vi "FineContrast_v3.0.vi"(3 "Contrast References":T4, 4 "Constrast Handles":T5, 5 "Scan Translation Exp Params":T2, 6 "Scan Translation Params":T6) -> (0 "Constrast Handles Out":T3, 1 "PZAPos & InstPow":dbl[][](array[numeric]), 2 "Spectra vs PZA":i32[][](array[numeric]))   [LabVIEW 2019]
uses:
  C:/Users/manip/Documents/Controle_Manip_2020/Thorlabs.MotionControl.KCube.SolenoidCLI.dll
  Thorlabs.MotionControl.KCube.SolenoidCLI.dll
  Light Field/lightfield-automation-labview/LightField Automation.lvclass
  TypeDefs/AcqMode.ctl
panel:
  out "KCube Shutter On?":bool
  out "range":dbl
  out "LinT End pos (mm)":dbl
  out "LinT Step Pos (mm)":dbl
  out "LinT Start Pos (mm)":dbl
  in  "ESP 301 error out":errorcluster
  in  "ESP 301 COM out":refnum<visa-resource-name>="COM1"
  out "ESP 301 error in":errorcluster
  out "ESP 301 COM":refnum<visa-resource-name>="COM1"
  in  "Photodiode error out":errorcluster {"code" format="%.0x"}
  out "Photodiode out":refnum<visa-resource-name>
  out "Scan Contrast Ctrls":refnum<vi>[](array[refnum])
  out "InstPow":dbl[](array[numeric])
  out "ExcPow_uW":dbl
  in  "ExcWL_nm":dbl
  out "Photodiode error in":errorcluster {"code" format="%.0x"}
  out "Photodiode in":refnum<visa-resource-name>
  out "WavelengthCalibration":dbl[](array[numeric])
  out "x+y":dbl
  out "Contrast Oscillations":refnum<vi>
  out "Contrast 1D Spectrum":refnum<vi>
  out "PZC out":string
  out "PZC error out":errorcluster
  out "Pause button":refnum<vi>
  in  "Stop button":refnum<vi>
  out "PZC Pos (usteps)":refnum<vi>
  out "PZA Positions":i32[](array[numeric])
  out "Contrast values":i32[](array[numeric])
  out "Contrast 1D Spectrum":cluster{dbl[], dbl[]}(graph) caption="64.0°"
  out "Contrast Oscillations":cluster{dbl[], dbl[]}(graph)
  out "LFA error out":errorcluster
  out "LFA out":refnum<class "LightField Automation.lvclass">
  in  "Acq Mode":T1=enum."Spectrum" caption="Mode :"
  in  "Acq Time (ms) 2":dbl=500.0 caption="Acq Time :" min=0.0 max=360000.0 step=50.0
  in  "Pause Contrast":bool
  in  "Stop Contrast":bool
  out "PZC Position Readout (usteps)":dbl caption="Readout (usteps)" min=-8.0 max=392.0
  out "Progess Bar":refnum<vi>
  out "Scan Spectrum Progess Bar":u8(slide) scale=0.0..100.0
  in  "LFA error in":errorcluster
  in  "LFA in":refnum<class "LightField Automation.lvclass">
  out "Shutter Device":refnum<vi>
  out "KCube Shutter Device Reference":refnum<k24>
  out "Shutter":refnum<vi>
  out "Shutter Ctrls":u16(ring)
  in  "CCD ROI":T7(ring)
  in  "Accumulations":dbl=1.0
  in  "LinTFine Step":dbl
  in  "LinTFine End":dbl
  in  "LinTFine Start":dbl
  # "ms"
types:
  T1 = typedef "AcqMode.ctl" = enum16{"Image", "Spectrum", "APD 1", "APD 2", "APD 1+2"}
  T2 = cluster{"Exposure Time (ms)":dbl, "Accumulations":dbl, "Excitation Wavelength (nm)":dbl, "Acq Mode":T1, "CCD ROI":enum16{"Custom ROI", "Full sensor", "Binned full sensor"}, "KCube Shutter On?":bool}
  T3 = cluster{"LightField Automation out":refnum<class "LightField Automation.lvclass">, "error out":errorcluster, "Instrument Channel out":string, "error out":errorcluster, "ESP 301 COM out":refnum<visa-resource-name>, "ESP 301 error out":errorcluster, "Photodiode out":refnum<visa-resource-name>, "Photodiode error out":errorcluster}
  T4 = cluster{"Shutter Ctrls":refnum<vi>, "KCube Shutter Device Reference":refnum<vi>, "Scan Main Progess Bar":refnum<vi>, "PZC Position Readout (usteps)":refnum<vi>, "Pause Contrast":refnum<vi>, "Stop Contrast":refnum<vi>, "Contrast 1D Spectrum":refnum<vi>, "Contrast Oscillations":refnum<vi>, "Acquire Contrast":refnum<vi>, "Save Contrast":refnum<vi>}
  T5 = cluster{"LightField Automation out":refnum<class "LightField Automation.lvclass">, "LightField Automation error out":errorcluster, "PZC200 Instrument Channel":string, "PZC Error":errorcluster, "ESP 301 COM Port":refnum<visa-resource-name>, "ESP 301 Error":errorcluster, "Photodiode handle out":refnum<visa-resource-name>, "Photodiode error out":errorcluster}
  T6 = cluster{"LinT Start Pos (mm)":dbl, "LinT Step Pos (mm)":dbl, "LinT End pos (mm)":dbl, "LinTFine Start Pos (usteps)":dbl, "LinTFines Step Pos (usteps)":dbl, "LinTFine End Pos (usteps)":dbl}
  T7 = enum16{"Custom ROI", "Full sensor", "Binned full sensor"}
  T8 = enum16{"Contrast", "Spectre", "Polarisation", "Time Trace", "XY Intensity Map"}
  T9 = enum16{"Image", "Spectrum", "APD 1", "APD 2", "APD 1+2"}
  T10 = cluster{"Image":dbl[][][], "Frame Size":cluster{"F":i32, "Y":i32, "X":i32}}[]
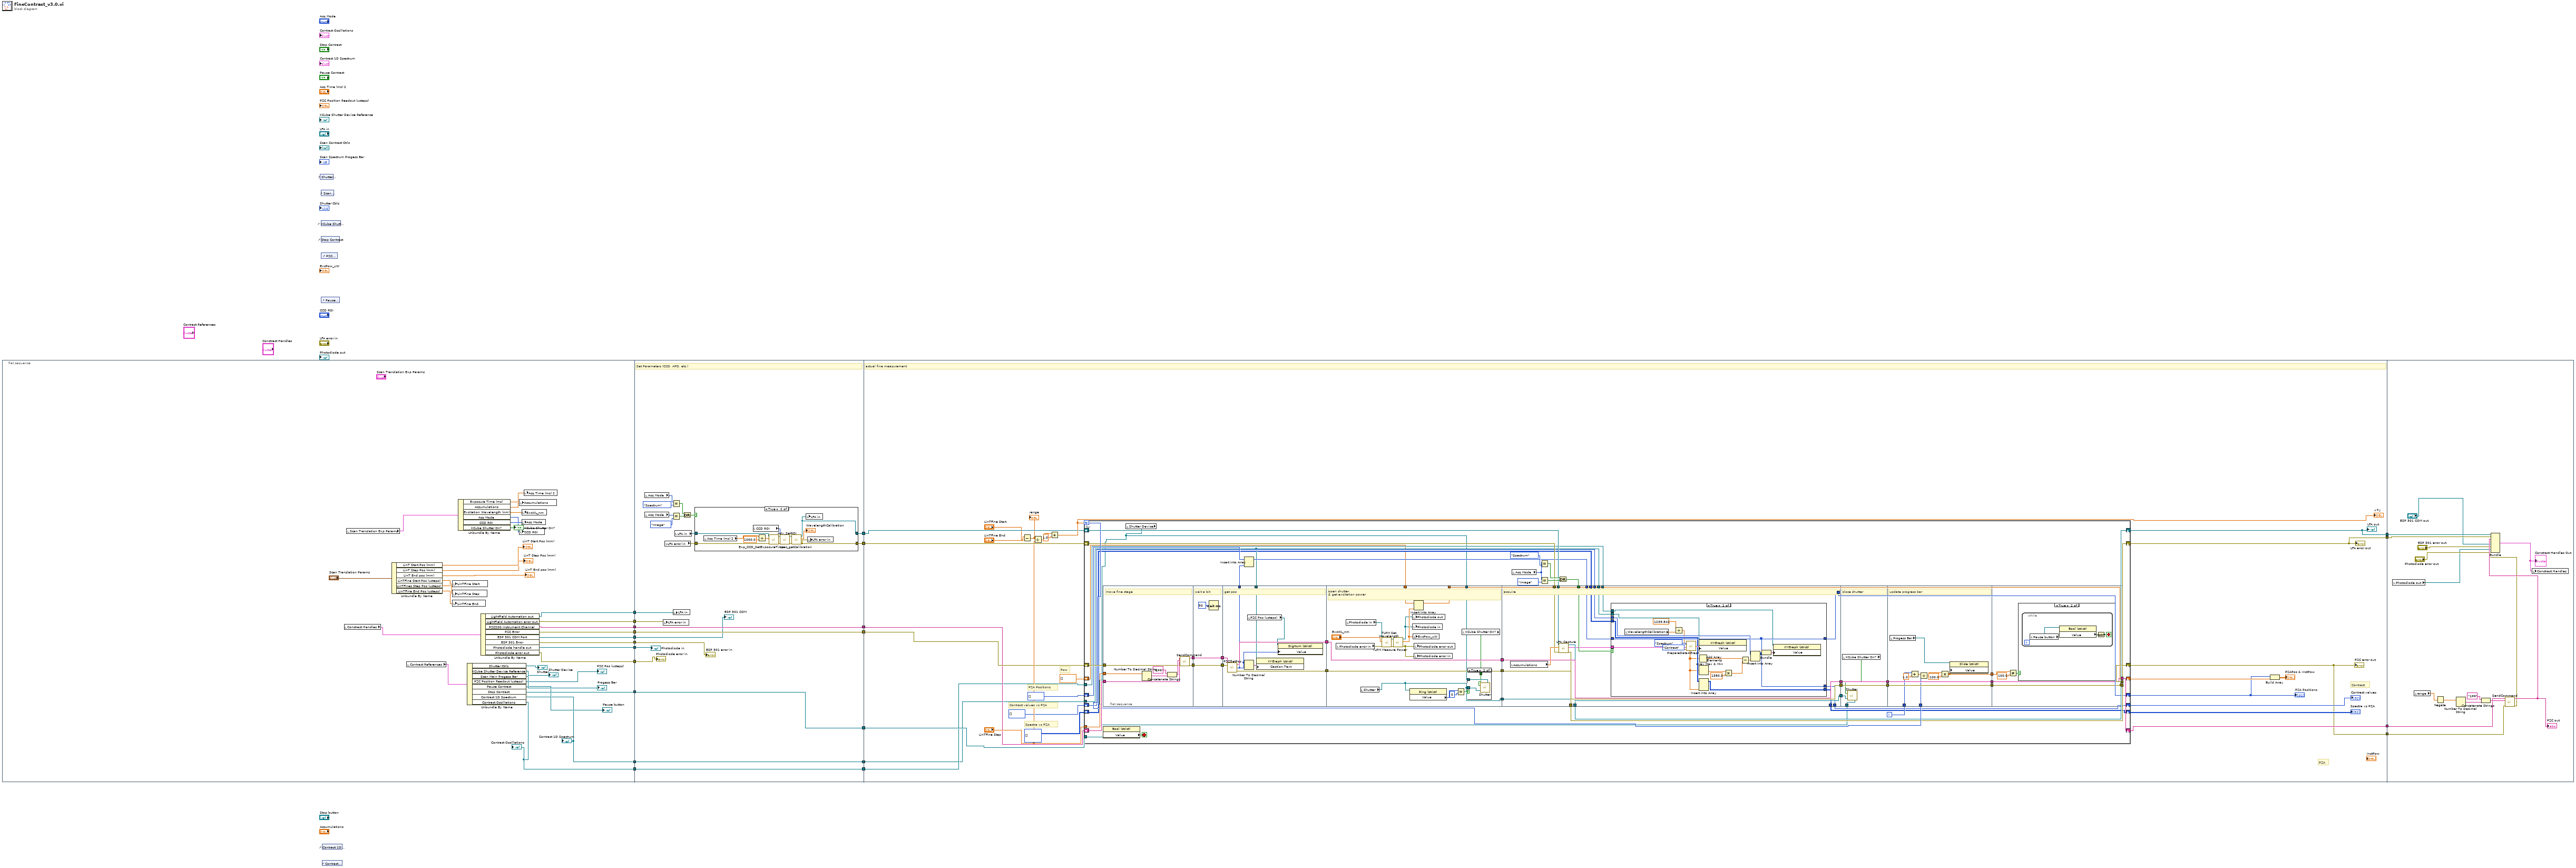
[diagram p0: block diagram]
diagram:
  n1 = flat-sequence {
    tunnel: [w41] -> w19
    tunnel: [w40] -> w18
    tunnel: [w38] -> w16
    tunnel: [w37] -> w14
    tunnel: [w36] -> w13
    tunnel: [w35] -> w12
    tunnel: [w34] -> w11
    tunnel: [w33] -> w10
    tunnel: [w31] -> w9
    tunnel: [w27] -> w6
    tunnel: [w26] -> w4
    tunnel: [w69] -> w22
    tunnel: [w68] -> w21
    tunnel: w19 -> [w65]
    tunnel: w18 -> [w64]
    tunnel: [w63] -> w17
    tunnel: w16 -> [w63]
    tunnel: [w62] -> w15
    tunnel: w14 -> [w62]
    tunnel: w13 -> [w61]
    tunnel: w12 -> [w60]
    tunnel: w11 -> [w59]
    tunnel: w10 -> [w58]
    tunnel: w9 -> [w57]
    tunnel: [w57] -> w8
    tunnel: [w56] -> w7
    tunnel: w6 -> [w56]
    tunnel: [w55] -> w5
    tunnel: w4 -> [w55]
    tunnel: w22 -> [w117]
    tunnel: w21 -> [w116]
    tunnel: [w100] -> w20
    tunnel: w17 -> [w99]
    tunnel: w15 -> [w98]
    tunnel: w8 -> [w97]
    tunnel: w7 -> [w96]
    tunnel: w5 -> [w95]
    tunnel: [w94] -> w3
    tunnel: [w93] -> w2
    tunnel: [w92] -> w1
    tunnel: w20 -> [w283]
    tunnel: w3 -> [w281]
    tunnel: w2 -> [w280]
    tunnel: w1 -> [w278]
    frame #0 {
      n2 = local read "Constrast Handles"() -> (w42:T5)
      n3 = local read "Scan Translation Exp Params"() -> (w24:T2)
      n4 = Unbundle By Name("Scan Translation Params") -> ("LinT Start Pos (mm)"=→"LinT Start Pos (mm)":dbl, "LinT Step Pos (mm)"=→"LinT Step Pos (mm)":dbl, "LinT End pos (mm)"=→"LinT End pos (mm)":dbl, "LinTFine Start Pos (usteps)"=w52:dbl, "LinTFines Step Pos (usteps)"=w53:dbl, "LinTFine End Pos (usteps)"=w54:dbl)
      n5 = local read "Contrast References"() -> (w39:T4)
      n6 = local write "LinTFine Start"(w52) -> ()
      n7 = local write "LinTFine Step"(w53) -> ()
      n8 = local write "LinTFine End"(w54) -> ()
      n9 = Unbundle By Name(w24) -> ("Exposure Time (ms)"=w50:dbl, "Accumulations"=w49:dbl, "Excitation Wavelength (nm)"=w48:dbl, "Acq Mode"=w47:T1, "CCD ROI"=w46:T7, "KCube Shutter On?"=→"KCube Shutter On?":bool)
      n10 = Unbundle By Name(w39) -> ("Shutter Ctrls"=→"Shutter":refnum<vi>, "KCube Shutter Device Reference"=→"Shutter Device":refnum<vi>, "Scan Main Progess Bar"=→"Progess Bar":refnum<vi>, "PZC Position Readout (usteps)"=→"PZC Pos (usteps)":refnum<vi>, "Pause Contrast"=→"Pause button":refnum<vi>, "Stop Contrast"=w31:refnum<vi>, "Contrast 1D Spectrum"=w26:refnum<vi>, "Contrast Oscillations"=w27:refnum<vi>)
      "Contrast Oscillations" <- w27
      "Contrast 1D Spectrum" <- w26
      n11 = Unbundle By Name(w42) -> ("LightField Automation out"=w41:refnum<class "LightField Automation.lvclass">, "LightField Automation error out"=w40:errorcluster, "PZC200 Instrument Channel"=w37:string, "PZC Error"=w38:errorcluster, "ESP 301 COM Port"=w34:refnum<visa-resource-name>, "ESP 301 Error"=w33:errorcluster, "Photodiode handle out"=w36:refnum<visa-resource-name>, "Photodiode error out"=w35:errorcluster)
      n12 = local write "Accumulations"(w49) -> ()
      n13 = local write "CCD ROI"(w46) -> ()
      n14 = local write "ExcWL_nm"(w48) -> ()
      n15 = local write "Acq Mode"(w47) -> ()
      n16 = local write "Acq Time (ms) 2"(w50) -> ()
    }
    frame #1 {
      # "Set Parameters (CCD, APD, etc.)"
      n17 = local read "Acq Mode"() -> (w76:T1)
      n18 = local read "Acq Mode"() -> (w72:T1)
      n19 = local write "LFA error in"(w64) -> ()
      n20 = local read "LFA error in"() -> (w67:errorcluster)
      n21 = Equal?(x=w76, y=AcqMode."Spectrum" ("Acq Mode")) -> (x = y?=w74:bool)
      n22 = Equal?(x=w72, y=AcqMode."Image" ("Acq Mode")) -> (x = y?=w71:bool)
      n23 = local write "LFA in"(w65) -> ()
      n24 = local read "LFA in"() -> (w66:refnum<class "LightField Automation.lvclass">)
      n25 = Or(x=w74, y=w71) -> (x .or. y?=w70:bool)
      n26 = case shown="True" w70 {
        tunnel: [w78 w85] -> w69
        tunnel: [w77 w84] -> w68
        tunnel: w67 -> [w77 w89]
        tunnel: w66 -> [w78 w88]
        frame False {
        }
        frame True {
          n27 = local read "Acq Time (ms) 2"() -> (w82:dbl)
          n28 = local read "CCD ROI"() -> (w79:T7)
          n29 = Divide(x=w82, y=1000.0) -> (x/y=w80:dbl)
          n30 = call "Exp_CCD_SetExposureTime.vi"("error in (no error)"=w89, "Exposure Time (s)"=w80, "LightField Automation in"=w88) -> ("error out"=w90:errorcluster, "LightField Automation out"=w91:refnum<class "LightField Automation.lvclass">)  [unwired: 7 in]
          n31 = call "Adv_SetROI.vi"("error in (no error)"=w90, "ROI"=w79, "LightField Automation in"=w91) -> ("error out"=w86:errorcluster, "LightField Automation out"=w87:refnum<class "LightField Automation.lvclass">)  [unwired: 7 in]
          n32 = call "spec_getCalibration.vi"("error in (no error)"=w86, "LightField Automation in"=w87) -> ("error out"=w84:errorcluster, "ColumnCalibration"=→"WavelengthCalibration":dbl[], "LightField Automation out"=w85:refnum<class "LightField Automation.lvclass">)  [unwired: 7 in]
          n33 = local write "LFA in"(w85) -> ()
          n34 = local write "LFA error in"(w84) -> ()
        }
      }
      "Photodiode in" <- w61
      "Photodiode error in" <- w60
      "ESP 301 COM" <- w59
      "ESP 301 error in" <- w58
    }
    frame #2 {
      # "PZA Positions"
      # "Pow"
      # "Spectra vs PZA"
      # "Contrast values vs PZA"
      # "Contrast"
      # "PZA"
      # "actual fine measurement"
      n35 = Subtract(x="LinTFine End", y="LinTFine Start") -> (x-y=w108:dbl)
      "range" <- w108
      n36 = Divide(x=w108, y="LinTFine Step") -> (x/y=w107:dbl)
      n37 = Add(x=w107, y=1.0) -> (x+y=w118:dbl)
      "x+y" <- w118
      n38 = for {
        N: w118 -> [w151]
        tunnel: "LinTFine Step" -> [w167]
        shift-right: [w146] -> w100
        shift-left: w98 -> [w165]
        shift-right: [w145] -> w92
        shift-left: w99 -> [w166]
        shift-right: [w135] -> w94
        shift-left: w117 -> [w137]
        shift-right: [w134] -> w93
        shift-left: w116 -> [w136]
        shift-right: [w124] -> w111
        shift-left: i32[] [] -> [w132]
        shift-right: [w123] -> w115
        shift-left: i32[] [] -> [w129]
        tunnel: w97 -> [w131]
        tunnel: w95 -> [w127]
        tunnel: w96 -> [w126]
        shift-right: [w122] -> w114
        shift-left: i32[][] [] -> [w125]
        shift-right: [w120] -> w113
        shift-left: dbl[] [] -> [w121]
        i -> [w152]
        stop <- w147 stop-if-true
        n39 = flat-sequence {
          tunnel: w167 -> [w175]
          tunnel: [w171] -> w164
          tunnel: [w170] -> w162
          tunnel: w166 -> [w169]
          tunnel: w165 -> [w168]
          tunnel: w164 -> [w178]
          tunnel: [w178] -> w163
          tunnel: w162 -> [w177]
          tunnel: [w177] -> w161
          tunnel: w163 -> [w186]
          tunnel: w161 -> [w185]
          tunnel: [w184] -> w160
          tunnel: [w183] -> w159
          tunnel: [w180] -> w133
          tunnel: w127 -> [w182]
          tunnel: w160 -> [w204]
          tunnel: w159 -> [w203]
          tunnel: w119 -> [w199]
          tunnel: [w204] -> w158
          tunnel: [w203] -> w157
          tunnel: [w188] -> w143
          tunnel: w121 -> [w193]
          tunnel: [w191] -> w120
          tunnel: w158 -> [w225]
          tunnel: w157 -> [w224]
          tunnel: [w225] -> w156
          tunnel: [w224] -> w155
          tunnel: [w222] -> w144
          tunnel: w143 -> [w222]
          tunnel: w137 -> [w221]
          tunnel: w136 -> [w220]
          tunnel: [w219] -> w135
          tunnel: [w218] -> w134
          tunnel: w130 -> [w217]
          tunnel: w129 -> [w215]
          tunnel: w128 -> [w214]
          tunnel: w127 -> [w213]
          tunnel: w126 -> [w212]
          tunnel: w125 -> [w211]
          tunnel: [w210] -> w124
          tunnel: [w209] -> w123
          tunnel: [w208] -> w122
          tunnel: w156 -> [w254]
          tunnel: w155 -> [w253]
          tunnel: [w254] -> w154
          tunnel: [w253] -> w153
          tunnel: w144 -> [w252]
          tunnel: w119 -> [w251]
          tunnel: w154 -> [w264]
          tunnel: w153 -> [w263]
          tunnel: w152 -> [w258]
          tunnel: w151 -> [w257]
          tunnel: [w264] -> w150
          tunnel: [w263] -> w149
          tunnel: [w256] -> w148
          tunnel: [w265] -> _
          tunnel: [w269] -> w146
          tunnel: w150 -> [w269]
          tunnel: w149 -> [w265]
          tunnel: w148 -> [w267]
          tunnel: [w265] -> w145
          frame #0 {
            # "move fine stage"
            n40 = Number To Decimal String(number=w175) -> (decimal integer string=w173:string)  [unwired: 1 in]
            n41 = Concatenate Strings("1PR", w173) -> (w172:string)
            n42 = call "SendCommand.vi"("error in"=w169, "Command"=w172, "Instrument Channel"=w168) -> ("error out"=w170:errorcluster, "Instrument Channel out"=w171:string)  [unwired: 7 in]
          }
          frame #1 {
            # "wait a bit"
            n43 = Wait (ms)(milliseconds to wait=u32 50) -> ()  [unwired: 1 out]
          }
          frame #2 {
            # "get pos"
            n44 = call "PZCGetPos.vi"("error in"=w185, "Instrument Channel"=w186) -> ("Instrument Channel Out"=w184:string, "Position"=w180:i32, "error out"=w183:errorcluster)
            n45 = Number To Decimal String(number=w180) -> (decimal integer string=w181:string)  [unwired: 1 in]
            n46 = local read "PZC Pos (usteps)"() -> (w179:refnum<vi>)
            n47 = property class="XYGraph (strict)"(reference=w182, "Caption.Text"=w181) -> ()  [unwired: 1 in, 2 out]
            n48 = property class="DigNum (strict)"(reference=w179, "Value"=w180) -> ()  [unwired: 1 in, 2 out]
          }
          frame #3 {
            # "open shutter\n& get excitation power"
            n49 = local read "Photodiode error in"() -> (w196:errorcluster)
            n50 = local read "Photodiode in"() -> (w195:refnum<visa-resource-name>)
            n51 = local read "Shutter"() -> (w188:refnum<vi>)
            n52 = call <instrlib>:"TLPM Set Wavelength.vi"("error in (no error)"=w196, "Wavelength (0.0)"="ExcWL_nm", "instrument handle"=w195) -> ("error out"=w197:errorcluster, "instrument handle out"=w198:refnum<visa-resource-name>)  [unwired: 7 in]
            n53 = call <instrlib>:"TLPM Measure Power.vi"("error in (no error)"=w197, "instrument handle"=w198) -> ("error out"=w189:errorcluster, "Power"=w192:dbl, "instrument handle out"=w190:refnum<visa-resource-name>)  [unwired: 7 in]
            n54 = property class="Ring (strict)"(reference=w188) -> ("Value"=w200:u16)  [unwired: 1 in, 2 out]
            n55 = local write "Photodiode out"(w190) -> ()
            n56 = local write "Photodiode in"(w190) -> ()
            n57 = local write "ExcPow_uW"(w192) -> ()
            n58 = Insert Into Array(array=w193, new element=w192) -> (w191:dbl[])  [unwired: 1 in]
            n59 = local write "Photodiode error out"(w189) -> ()
            n60 = local write "Photodiode error in"(w189) -> ()
            n61 = Equal?(x=w200, y=u16 0) -> (x = y?=w201:bool)
            n62 = local read "KCube Shutter On?"() -> (w187:bool)
            n63 = case shown="True" w201 {
              tunnel: w188 -> [_ w207]
              tunnel: w199 -> [_ w206]
              tunnel: w187 -> [_ w205]
              frame False {
              }
              frame True {
                n64 = call "Shutter.vi"("KCube Shutter Device Reference 2"=w206, "Shutter Ctrls 2"=w207, "Shutter on?"=w205) -> ()
              }
            }
          }
          frame #4 {
            # "acquire"
            n65 = local read "Accumulations"() -> (w223:dbl)
            n66 = call "LFA_Capture.vi"("error in (no error)"=w220, "Frames"=w223, "LightField Automation in"=w221) -> ("error out"=w218:errorcluster, "Data"=w216:T10, "LightField Automation out"=w219:refnum<class "LightField Automation.lvclass">)  [unwired: 6 in]
            n67 = case shown="True" w217 {
              tunnel: w216 -> [_ w249]
              tunnel: w215 -> [w227 w248]
              tunnel: w214 -> [w228 w246]
              tunnel: [w228 w246] -> w210
              tunnel: [w227 w245] -> w209
              tunnel: w213 -> [_ w244]
              tunnel: w212 -> [_ w243]
              tunnel: w211 -> [w226 w240]
              tunnel: [w226 w239] -> w208
              frame False {
              }
              frame True {
                n68 = local read "WavelengthCalibration"() -> (w232:dbl[])
                n69 = Divide(x=1239.842, y=w232) -> (x/y=w230:dbl[])
                n70 = call "PrepareData4Graph.vi"("Wavelength nm"=w230, "DataLF"=w249, "AcqMode"=T9."Spectrum", "Data type"=T8."Contrast") -> ("Spectrum"=w241:cluster{"Array 2":dbl[], "Array":dbl[]}, "PLInt out"=w235:dbl[])  [unwired: 2 in, 3 out]
                n71 = Add Array Elements(numeric array=w235) -> (sum=w238:dbl)
                n72 = property class="XYGraph (strict)"(reference=w244, "Value"=w241) -> ()  [unwired: 1 in, 2 out]
                n73 = Array Max & Min(array=w235) -> (min value=w234:dbl)  [unwired: 3 out]
                n74 = Insert Into Array(array=w240, new element=w235) -> (w239:i32[][])  [unwired: 2 in]
                n75 = Multiply(x=w234, y=1380.0) -> (x*y=w233:dbl)
                n76 = Subtract(x=w238, y=w233) -> (x-y=w237:dbl)
                n77 = Insert Into Array(array=w248, new element=w237) -> (w245:i32[])  [unwired: 1 in]
                n78 = Bundle(w246, w245) -> (w247:cluster{i32[], i32[]})  [unwired: 1 in]
                n79 = property class="XYGraph (strict)"(reference=w243, "Value"=w247) -> ()  [unwired: 1 in, 2 out]
              }
            }
          }
          frame #5 {
            # "close shutter"
            n80 = local read "KCube Shutter On?"() -> (w250:bool)
            n81 = call "Shutter.vi"("KCube Shutter Device Reference 2"=w251, "Shutter Ctrls 2"=w252, "Shutter on?"=w250) -> ()
          }
          frame #6 {
            # "update progress bar"
            n82 = local read "Progess Bar"() -> (w255:refnum<vi>)
            n83 = Add(x=w258, y=1.0) -> (x+y=w261:dbl)
            n84 = Divide(x=w261, y=w257) -> (x/y=w260:dbl)
            n85 = Multiply(x=w260, y=100.0) -> (x*y=w256:dbl)
            n86 = property class="Slide (strict)"(reference=w255, "Value"=w256) -> ()  [unwired: 1 in, 2 out]
          }
          frame #7 {
            n87 = Not Equal?(x=w267, y=100.0) -> (x != y?=w266:bool)
            n88 = case shown="True" w266 {
              frame False {
              }
              frame True {
                n89 = while {
                  stop <- w271 stop-if-true
                  n90 = local read "Pause button"() -> (w270:refnum<vi>)
                  n91 = property class="Bool (strict)"(reference=w270) -> ("Value"=w272:bool)  [unwired: 1 in, 2 out]
                  n92 = Not(x=w272) -> (.not. x?=w271:bool)
                }
              }
            }
          }
        }
        n93 = property class="Bool (strict)"(reference=w131) -> ("Value"=w147:bool)  [unwired: 1 in, 2 out]
        n94 = local read "Shutter Device"() -> (w119:refnum<vi>)
        n95 = Insert Into Array(array=w132, new element=w133) -> (w128:i32[])  [unwired: 1 in]
        n96 = local read "Acq Mode"() -> (w142:T1)
        n97 = Equal?(x=w142, y=AcqMode."Spectrum" ("Acq Mode")) -> (x = y?=w138:bool)
        n98 = Equal?(x=w142, y=AcqMode."Image" ("Acq Mode")) -> (x = y?=w139:bool)
        n99 = Or(x=w138, y=w139) -> (x .or. y?=w130:bool)
      }
      "LFA out" <- w94
      "LFA error out" <- w93
      "Contrast values" <- w115
      "PZC error out" <- w92
      "Spectra vs PZA" <- w114
      "PZA Positions" <- w111
      n100 = Build Array(w111, w113) -> (→"PZAPos & InstPow":dbl[][])
    }
    frame #3 {
      n101 = local read "Photodiode out"() -> (w273:refnum<visa-resource-name>)
      n102 = local read "range"() -> (w286:dbl)
      n103 = Negate(x=w286) -> (-x=w285:dbl)
      n104 = Number To Decimal String(number=w285) -> (decimal integer string=w288:string)  [unwired: 1 in]
      n105 = Concatenate Strings("1PR", w288) -> (w287:string)
      n106 = call "SendCommand.vi"("error in"=w278, "Command"=w287, "Instrument Channel"=w283) -> ("error out"=w277:errorcluster, "Instrument Channel out"=w279:string)  [unwired: 7 in]
      "PZC out" <- w279
      n107 = Bundle("LightField Automation out"=w281, "error out"=w280, "Instrument Channel out"=w279, "error out"=w277, "ESP 301 COM out"="ESP 301 COM out", "ESP 301 error out"="ESP 301 error out", "Photodiode out"=w273, "Photodiode error out"="Photodiode error out") -> (w282:T3)  [unwired: 1 in]
      "Constrast Handles Out" <- w282
      n108 = local write "Constrast Handles"(w282) -> ()
    }
  }
  n109 = control-ref of="Shutter Ctrls"() -> ()  [unwired: 1 out]
  n110 = control-ref of="Scan Spectrum Progess Bar"() -> ()  [unwired: 1 out]
  n111 = control-ref of="KCube Shutter Device Reference"() -> ()  [unwired: 1 out]
  n112 = control-ref of="Stop Contrast"() -> ()  [unwired: 1 out]
  n113 = control-ref of="PZC Position Readout (usteps)"() -> ()  [unwired: 1 out]
  n114 = control-ref of="Pause Contrast"() -> ()  [unwired: 1 out]
  n115 = control-ref of="Contrast 1D Spectrum"() -> ()  [unwired: 1 out]
  n116 = control-ref of="Contrast Oscillations"() -> ()  [unwired: 1 out]
